vi "svl_Equivalent Continuous Level with IC_octave.vi"(2 "init/cont (init:F)":bool, 3 "initial internal state":cluster{"squared sum":dbl, "size":dbl} {"size" format="%.2f"; "squared sum" format="%.2f"}, 4 "scaled signal [EU]":dbl[](array[numeric]) format="%.2f") -> (0 "final internal state":cluster{"squared sum":dbl, "size":dbl} {"size" format="%.2f"; "squared sum" format="%.2f"}, 1 "equivalent continuous level [EU^2 rms]":dbl format="%.2f")   [LabVIEW 2017]
doc: "Computes the equivalent continuous level of the input signal.\nThe initial internal state and final internal state keep track of the internal state of the averaging process to ensure continuous operation if you use continuous mode."
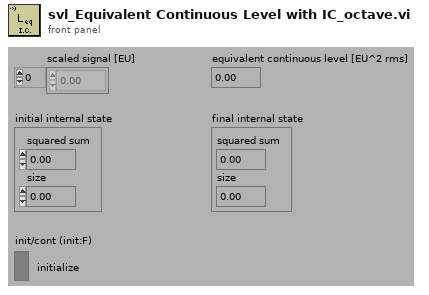
[diagram p1: front panel]
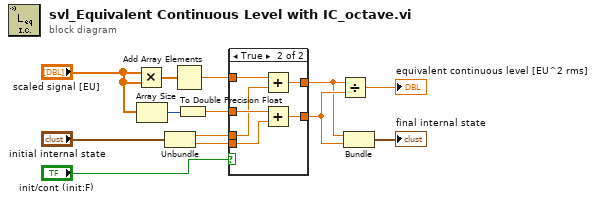
[diagram p0: block diagram]
diagram:
  n1 = Multiply(x="scaled signal [EU]", y="scaled signal [EU]") -> (x*y=w2:dbl[])
  n2 = Array Size(array="scaled signal [EU]") -> (size(s)=w13:i32)
  n3 = Unbundle("initial internal state") -> ("squared sum"=w9:dbl, "size"=w8:dbl)
  n4 = Add Array Elements(numeric array=w2) -> (sum=w3:dbl)
  n5 = To Double Precision Float(number=w13) -> (double precision float=w10:dbl)
  n6 = case shown="True" "init/cont (init:F)" {
    tunnel: w3 -> [w15 w18]
    tunnel: w10 -> [w14 w21]
    tunnel: [w14 w20] -> w7
    tunnel: [w15 w19] -> w6
    tunnel: w9 -> [_ w17]
    tunnel: w8 -> [_ w16]
    frame False {
    }
    frame True {
      n7 = Add(x=w18, y=w17) -> (x+y=w19:dbl)
      n8 = Add(x=w21, y=w16) -> (x+y=w20:dbl)
    }
  }
  n9 = Divide(x=w6, y=w7) -> (x/y=→"equivalent continuous level [EU^2 rms]":dbl)
  n10 = Bundle(w6, w7) -> (→"final internal state":cluster{dbl, dbl})  [unwired: 1 in]
